vi "first try.vi"() -> ()   [LabVIEW 2017]
uses:
  <vilib>/rvi/Emulation/niFpgaGetClockAttributes.vi
  <vilib>/rvi/Emulation/niFpgaSctlEmulationGetInTimedLoop.vi
  <vilib>/rvi/Emulation/niFpgaEmulationReportErrorSimple.vi
  <vilib>/rvi/eio/common/nirviEmuTemplateMethod_errors.vi
  <vilib>/rvi/Emulation/niFpgaCriticalErrorInLSC.vi
  <vilib>/eio/EIOMethodNode/EIOMethodNode.xnode
  <vilib>/eio/EIONode/EIONode.xnode
panel:
  in  "stop 2":bool
  in  "I/O Item 2":bool
  in  "stop":bool
  out "I/O Item":bool
  in  "Enable":bool
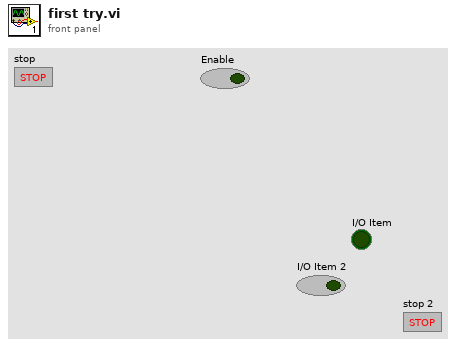
[diagram p1: front panel]
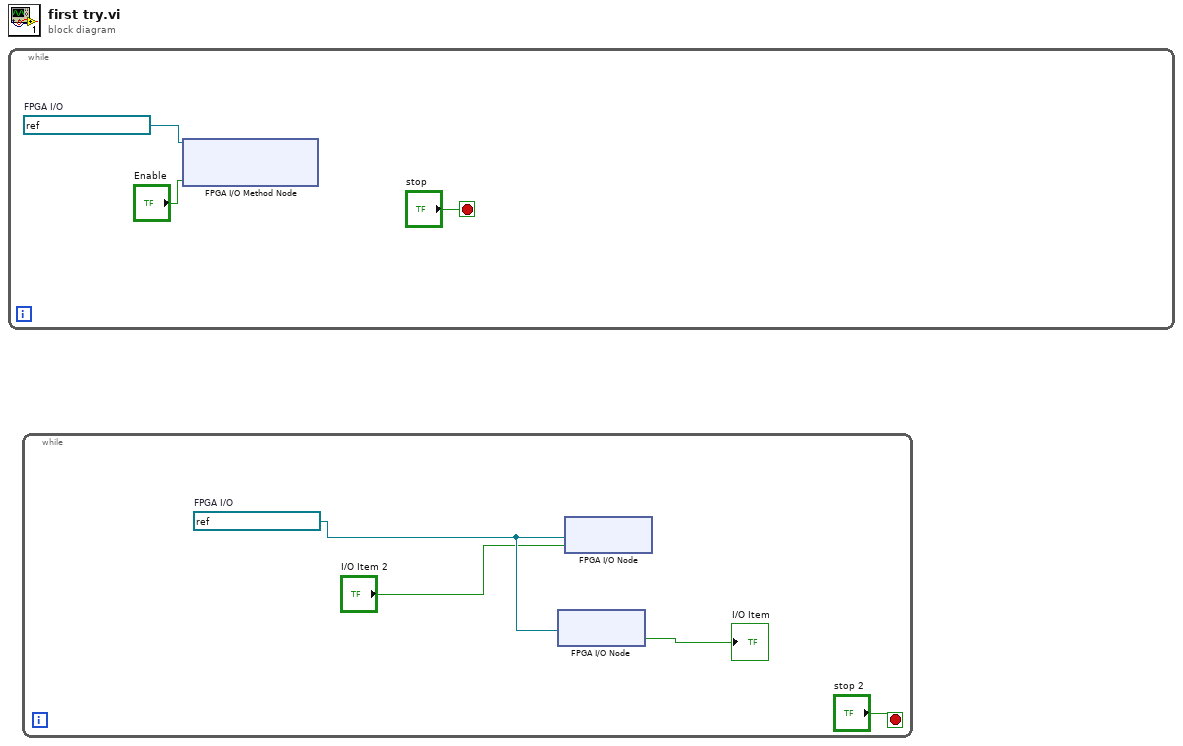
[diagram p0: block diagram]
diagram:
  n1 = while {
    stop <- "stop" stop-if-true
    w2 = refnum<k21> "Connector0/DIO25"  # FPGA I/O
    n2 = xnode "FPGA I/O Method Node"("FPGA I/O In"=w2, "Enable"="Enable") -> ()  [unwired: 1 out]
  }
  n3 = while {
    stop <- "stop 2" stop-if-true
    w6 = refnum<k21> "Connector0/DIO25"  # FPGA I/O
    n4 = xnode "FPGA I/O Node"("FPGA I/O In"=w6) -> ("I/O Item"=→"I/O Item":bool)  [unwired: 1 out]
    n5 = xnode "FPGA I/O Node"("I/O Item"="I/O Item 2", "FPGA I/O In"=w6) -> ()  [unwired: 1 out]
  }
